vi "Get message from save image VI.vi"(8 "error in (no error)":errorcluster, 11 "Channel in":refnum<class "SPARC4_Channel.lvclass">) -> (0 "error out":errorcluster, 3 "Channel out":refnum<class "SPARC4_Channel.lvclass">)   [LabVIEW 2018, in "SPARC4_Channel.lvclass"]
doc: "Get message from the save image VI"
uses:
  SPARC4_Channel.lvclass
  SPARC4_Channel.lvclass/SPARC4_Channel.ctl
  RxTx/RxTx.lvclass
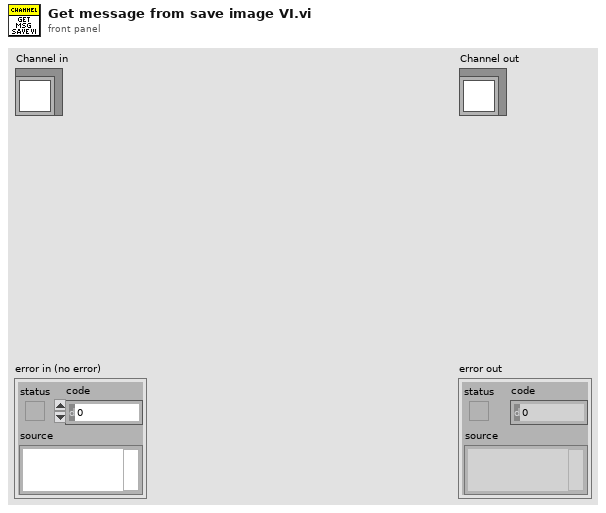
[diagram p1: front panel]
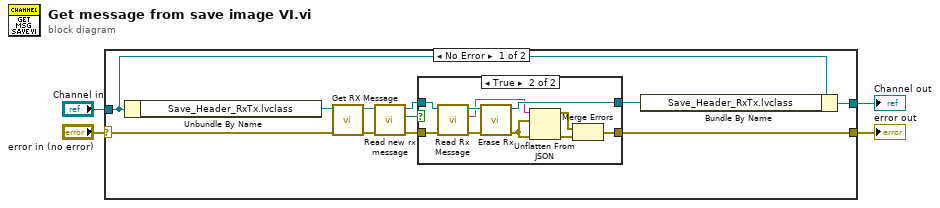
[diagram p0: block diagram]
diagram:
  n1 = case shown="No Error" "error in (no error)" {
    selector: "error in (no error)" -> [w13 w29]
    tunnel: [w11 w29] -> w3
    tunnel: [w10 w28] -> w1
    tunnel: "Channel in" -> [w15 w28]
    frame No Error {
      n2 = Unbundle By Name(w15) -> ("Save_Header_RxTx.lvclass"=w14:refnum<class "RxTx.lvclass">)
      n3 = call "Get RX Message.vi"("error in (no error)"=w13, "RxTx in"=w14) -> ("error out"=w9:errorcluster, "RxTx out"=w6:refnum<class "RxTx.lvclass">)  [unwired: 8 in]
      n4 = call-dynamic "Read new rx message.vi"("error in (no error)"=w9, "RxTx in"=w6) -> ("error out"=w8:errorcluster, "new rx message"=w5:bool, "RxTx out"=w7:refnum<class "RxTx.lvclass">)  [unwired: 7 in]
      n5 = case shown="True" w5 {
        tunnel: w8 -> [w16 w26]
        tunnel: w7 -> [w17 w27]
        tunnel: [w17 w21] -> w12
        tunnel: [w16 w18] -> w11
        frame False {
        }
        frame True {
          n6 = call "Read Rx Message.vi"("error in (no error)"=w26, "RxTx in"=w27) -> ("error out"=w23:errorcluster, "Rx Message"=w19:string, "RxTx out"=w22:refnum<class "RxTx.lvclass">)  [unwired: 7 in]
          n7 = call "Erase Rx.vi"("error in (no error)"=w23, "RxTx in"=w22) -> ("error out"=w20:errorcluster, "RxTx out"=w21:refnum<class "RxTx.lvclass">)  [unwired: 8 in]
          n8 = Unflatten From JSON(JSON string=w19, type and defaults=w20, error in (no error)=w20) -> (value=w24:errorcluster, error out=w25:errorcluster)  [unwired: 4 in]
          n9 = Merge Errors(w24, w25) -> (w18:errorcluster)
        }
      }
      n10 = Bundle By Name(cluster=w15, "Save_Header_RxTx.lvclass"=w12) -> (w10:refnum<class "SPARC4_Channel.lvclass">)
    }
    frame Error {
    }
  }
  "error out" <- w3
  "Channel out" <- w1
